vi "Read Headers.vi"(7 "Linked List ID":string, 8 "error in (no error)":errorcluster, 11 "Linked List in":refnum<class "Linked List.lvclass">) -> (0 "error out":errorcluster, 1 "Header Values":string[](array[string]), 2 "Header Names":string[](array[string]), 3 "Linked List out":refnum<class "Linked List.lvclass">, 4 "found":bool)   [LabVIEW 2020, in "Linked Lists.lvlib" / "Linked List.lvclass"]
uses:
  <vilib>/gpm_packages/@cs/linked-list/Source/Linked List/Linked List/Linked List.lvclass
  <vilib>/gpm_packages/@cs/linked-list/Source/Linked List/Linked List Definition/Linked List Definition.lvclass
  <vilib>/gpm_packages/@cs/linked-list/Source/Linked List/Linked List/Linked List.lvclass/Linked List.ctl
  <vilib>/gpm_packages/@cs/lookup-table/Source/LookupTable/LookupTable.lvclass/LookupTable.ctl
  e6b6f11a-f4b1-429b-bf9e-268286b052e2.vi
  <vilib>/gpm_packages/@cs/lookup-table/Source/LookupTable/Read Table Reference.vi
  e6b6f11a-f4b1-429b-bf9e-268286b052e2.vi/5a7267ad-595e-4610-9ac2-8bef780848ff.vi
  <vilib>/gpm_packages/@cs/lookup-table/Source/LookupTable/LookupTable.lvclass
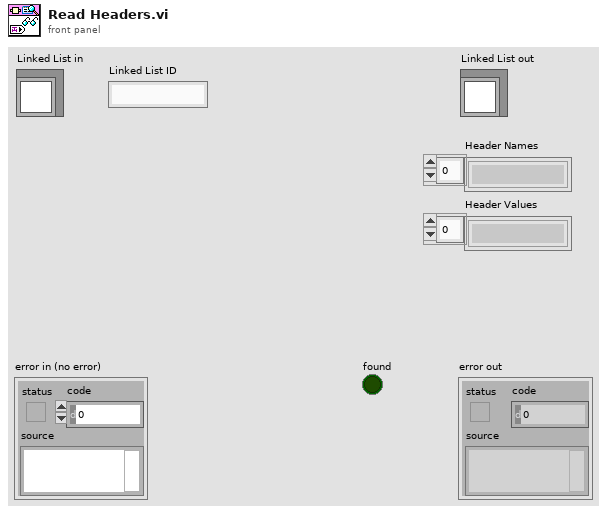
[diagram p1: front panel]
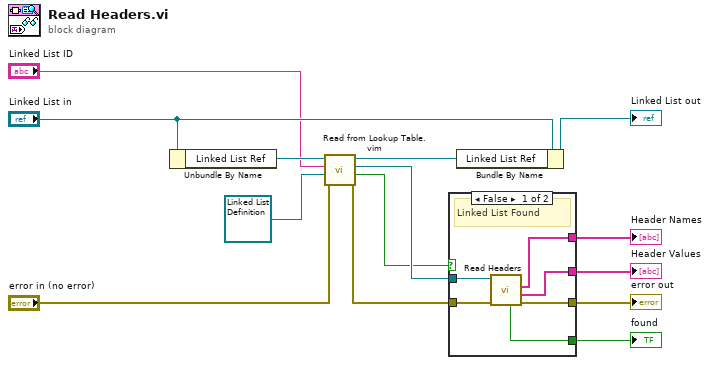
[diagram p0: block diagram]
diagram:
  n1 = Unbundle By Name("Linked List in") -> ("Linked List Ref"=w14:refnum<data-value>)
  n2 = call "Read from Lookup Table.vim"("error in (no error)"="error in (no error)", "Type"=refnum<class "Linked List Definition.lvclass"> refnum ("Linked List.lvlib:Linked List Definition.lvclass"), "Item Name"="Linked List ID", "LookupTable Reference"=w14) -> ("error out"=w11:errorcluster, "Not Found?"=w9:bool, "Value"=w10:refnum<class "Linked List Definition.lvclass">, "LookupTable Reference Out"=w12:refnum<data-value>)  [unwired: 4 in]
  n3 = case shown="False" w9 {
    tunnel: w11 -> [w20 w21]
    tunnel: [w19 w21] -> w7
    tunnel: w10 -> [w18 _]
    tunnel: [w17 _] -> w3
    tunnel: [w16 _] -> w2
    tunnel: [w15 _] -> w1
    frame False {
      # "Linked List Found"
      n4 = call <vilib>:"Read Headers.vi"("error in (no error)"=w20, "Linked List Definition in"=w18) -> ("error out"=w19:errorcluster, "Header Values"=w16:string[], "Header Names"=w15:string[], "Found?"=w17:bool)  [unwired: 5 in, 1 out]
    }
    frame True {
      # "Linked List not found"
    }
  }
  "error out" <- w7
  "Header Values" <- w2
  "Header Names" <- w1
  "found" <- w3
  n5 = Bundle By Name(cluster="Linked List in", "Linked List Ref"=w12) -> (→"Linked List out":refnum<class "Linked List.lvclass">)
